vi "Open Session.vi"(8 "error in":errorcluster, 11 "SessionOptions":T1) -> (0 "error out":errorcluster, 1 "Opened":bool, 2 "Session Ref":refnum<k24>)   [LabVIEW 2015, in "LV-WinSCP.lvlib"]
uses:
  LV-WinSCP.lvlib
  SessionOptions Ref.ctl
  C:/Program Files (x86)/WinSCP/WinSCPnet.dll
  Program Files (x86)/WinSCP/WinSCPnet.dll
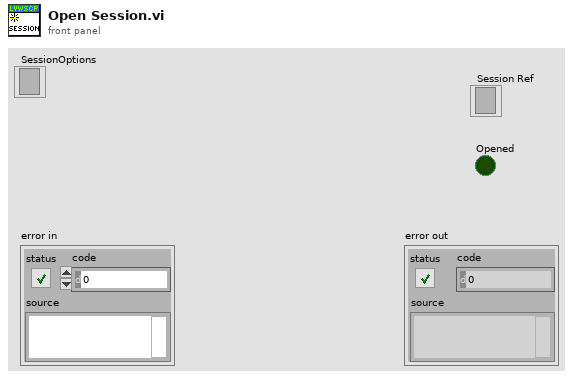
[diagram p1: front panel]
types:
  T1 = typedef "LV-WinSCP.lvlib/SessionOptions Ref.ctl" = refnum<k24>
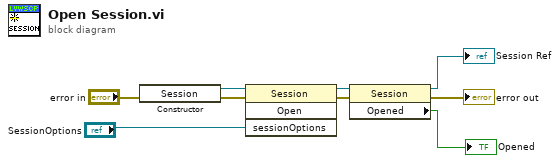
[diagram p0: block diagram]
diagram:
  n1 = constructor class="Session"(error in="error in") -> (reference out=w9:refnum<k24>, error out=w8:errorcluster)  [unwired: 2 in, 1 out]
  n2 = invoke class="Session" method="Open"(reference=w9, error in=w8, "sessionOptions"="SessionOptions") -> (reference out=w5:refnum<k24>, error out=w4:errorcluster)  [unwired: 1 in, 2 out]
  n3 = property class="Session"(reference=w5, error in=w4) -> (reference out=→"Session Ref":refnum<k24>, error out=→"error out":errorcluster, "Opened"=→"Opened":bool)
